vi "Variant to String.vi"(8 "error in (no error)":errorcluster, 11 "Data (Variant)":variant) -> (0 "error out":errorcluster, 3 "Value":string)   [LabVIEW 2019, in "Data.lvclass"]
uses:
  Data.lvclass
  <vilib>/Utility/Data Type/NI_Data Type.lvlib
  <vilib>/ErrorRing/Error Ring.xnode
  <vilib>/Utility/error.llb/Error Cluster From Error Code.vi
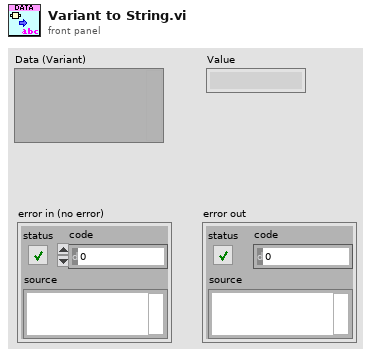
[diagram p1: front panel]
types:
  T1 = typedef "NI_Data Type.lvlib/Data Type.ctl" = enum8{"Invalid Type", "Void", "I8", "I16", "I32", "I64", "U8", "U16", "U32", "U64", "Single Float", "Double Float", "Extended Float", "Single Complex", "Double Complex", "Extended Complex", "Enum U8", "Enum U16", "Enum U32", "Enum U64", "Single Float With Unit", "Double Float With Unit", "Extended Float With Unit", "Single Complex with Unit", "Double Complex with Unit", "Extended Complex with Unit", "Boolean", "String", "Path", "Picture", "Tag", "Array", "Cluster", "Variant", "LV Variant", "Waveform", "Timestamp", "Digital Waveform", "Digital Data", "ExpressData", "Refnum", "External Data", "VI", "Poly VI", "LabVIEW Class Instance", "Fixed Point", "Set Collection", "Map Collection"}
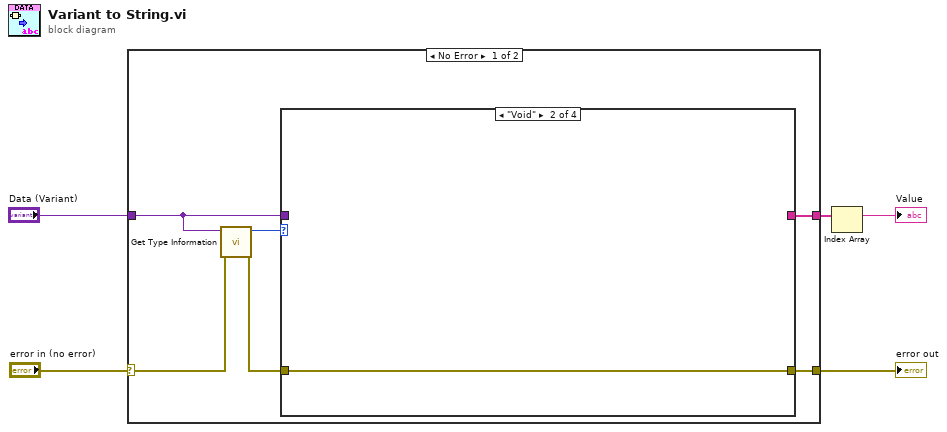
[diagram p0: block diagram]
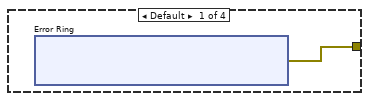
[diagram p2: hidden frame]
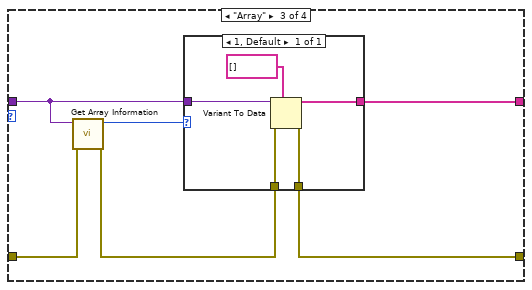
[diagram p3: hidden frame]
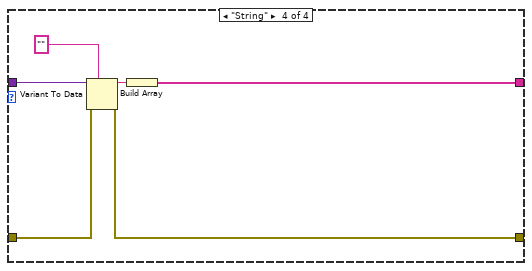
[diagram p4: hidden frame]
diagram:
  n1 = case shown="No Error" "error in (no error)" {
    selector: "error in (no error)" -> [w6 w35]
    tunnel: [w10 _] -> w2
    tunnel: [w7 w35] -> w5
    tunnel: "Data (Variant)" -> [w9 _]
    frame No Error {
      n2 = call <vilib>:"Get Type Information.vi"("error in (no error)"=w6, "variant"=w9) -> ("error out"=w8:errorcluster, "type"=w11:T1)  [unwired: 5 in, 3 out]
      n3 = case shown="\"Void\"" w11 {
        tunnel: [w12 w17 w23 w30] -> w7
        tunnel: [_ _ w18 w32] -> w10
        tunnel: w9 -> [_ _ w22 w33]
        tunnel: w8 -> [_ w17 w21 w31]
        frame Default {
          n4 = xnode "Error Ring"() -> ("error out"=w12:errorcluster)
        }
        frame "Void" {
        }
        frame "Array" {
          n5 = call <vilib>:"Get Array Information.vi"("error in (no error)"=w21, "variant"=w22) -> ("error out"=w20:errorcluster, "number of dimensions"=w19:i32)  [unwired: 6 in, 2 out]
          n6 = case shown="1, Default" w19 {
            tunnel: [w27] -> w23
            tunnel: w22 -> [w26]
            tunnel: w20 -> [w25]
            tunnel: [w24] -> w18
            frame 1, Default {
              n7 = Variant To Data(error in=w25, type=string[] [], Variant=w26) -> (data=w24:string[], error out=w27:errorcluster)
            }
          }
        }
        frame "String" {
          n8 = Variant To Data(error in=w31, type="", Variant=w33) -> (data=w34:string, error out=w30:errorcluster)
          n9 = Build Array(w34) -> (w32:string[])
        }
      }
    }
    frame Error {
    }
  }
  "error out" <- w5
  n10 = Index Array(array=w2) -> (element=→"Value":string)  [unwired: 1 in]
